vi "performanceCalc.vi"(0 "errors":dbl[](array[numeric]), 1 "init":bool, 2 "windowLength":dbl, 5 "pckTotalTrack":dbl[](array[numeric]), 7 "state":dbl[](array[numeric]), 9 "pckSuccess":dbl, 11 "pckTotal":dbl, 12 "delay":dbl) -> (4 "errorsOut":dbl[](array[numeric]), 6 "pckTotalTrackOut":dbl[](array[numeric]), 8 "prevState":dbl[](array[numeric]))   [LabVIEW 2010]
uses:
  <vilib>/imath/engines/lvmath2/RunTimeEngine/ErrorHandling/NIMS_Finalize Error.vi
  <vilib>/imath/engines/lvmath2/RunTimeEngine/VariableToken/Read/NIMS_Get Elements - RV(_) - Check.vi
  <instcachedir>/0/NIMS_Get Elements - RV(_) - Check_1F6F8656162345078B1D4DC9877DFAE9.lvgen/NIMS_Get Elements - RV(_) - Check_1F6F8656162345078B1D4DC9877DFAE9_000.vi
  <vilib>/imathl/engines/lvmath/Functions/Error Handling/Create Error.vi
  <vilib>/imath/engines/lvmath2/RunTimeEngine/NodeEndStatement/NIMS_NodeEndStatement_Output.vi
  <instcachedir>/0/NIMS_NodeEndStatement_Output_53EC0D466D134D7ABD903AC30B43404B.lvgen/NIMS_NodeEndStatement_Output_53EC0D466D134D7ABD903AC30B43404B_001.vi
  <instcachedir>/0/NIMS_NodeEndStatement_Output_53EC0D466D134D7ABD903AC30B43404B.lvgen/NIMS_NodeEndStatement_Output_53EC0D466D134D7ABD903AC30B43404B_005.vi
  <vilib>/imath/engines/lvmath2/RunTimeEngine/BuiltInFunctions/mod/NIMS_mod_no_size_check.vi
  <instcachedir>/0/NIMS_mod_no_size_check_5393E3382FD241D281EEB71DA286C65B.lvgen/NIMS_mod_no_size_check_5393E3382FD241D281EEB71DA286C65B_001.vi
  <vilib>/imath/engines/lvmath2/RunTimeEngine/ReplaceToken/NIMS_Replace - Check(_) Linear.vi
  <instcachedir>/0/NIMS_Replace - Check(_) Linear_D531E313C4004E3DB8F0EA3CE86AE758.lvgen/NIMS_Replace - Check(_) Linear_D531E313C4004E3DB8F0EA3CE86AE758_006.vi
  <vilib>/imath/engines/lvmath2/RunTimeEngine/ReplaceToken/NIMS_Replace - Size Check _(_)=S.vi
  <instcachedir>/0/NIMS_Replace - Size Check _(_)=S_6CAC13ACC74349C582FDAB09BCDAB70F.lvgen/NIMS_Replace - Size Check _(_)=S_6CAC13ACC74349C582FDAB09BCDAB70F_000.vi
  <vilib>/imath/engines/lvmath2/RunTimeEngine/ReplaceToken/NIMS_Replace - V(S)=S.vi
  <instcachedir>/0/NIMS_Replace - V(S)=S_78FDB6CCD265407D8926E4CF958018EB.lvgen/NIMS_Replace - V(S)=S_78FDB6CCD265407D8926E4CF958018EB_000.vi
  <vilib>/imath/engines/lvmath2/RunTimeEngine/VariableToken/Read/NIMS_Get Elements - RV(_) - Check(_).vi
  <instcachedir>/0/NIMS_Get Elements - RV(_) - Check(_)_260A45C9C4AF472A8F32F86A1BEF7DEE.lvgen/NIMS_Get Elements - RV(_) - Check(_)_260A45C9C4AF472A8F32F86A1BEF7DEE_000.vi
  <vilib>/imath/engines/lvmath2/RunTimeEngine/BuiltInFunctions/sum/NIMS_sum(GV).vi
  <instcachedir>/0/NIMS_sum(GV)_67F5EC36BC034E54A6BEC5B0673C00E5.lvgen/NIMS_sum(GV)_67F5EC36BC034E54A6BEC5B0673C00E5_000.vi
  <vilib>/imath/engines/lvmath2/RunTimeEngine/ReplaceToken/NIMS_Replace - Check Linear.vi
  <instcachedir>/0/NIMS_Replace - Check Linear_662D5651E4E34E0584DA82A256193A4C.lvgen/NIMS_Replace - Check Linear_662D5651E4E34E0584DA82A256193A4C_001.vi
  <vilib>/imath/engines/lvmath2/RunTimeEngine/ErrorHandling/NIMS_Create Error From Enums.vi
panel:
  out "interSampling":dbl
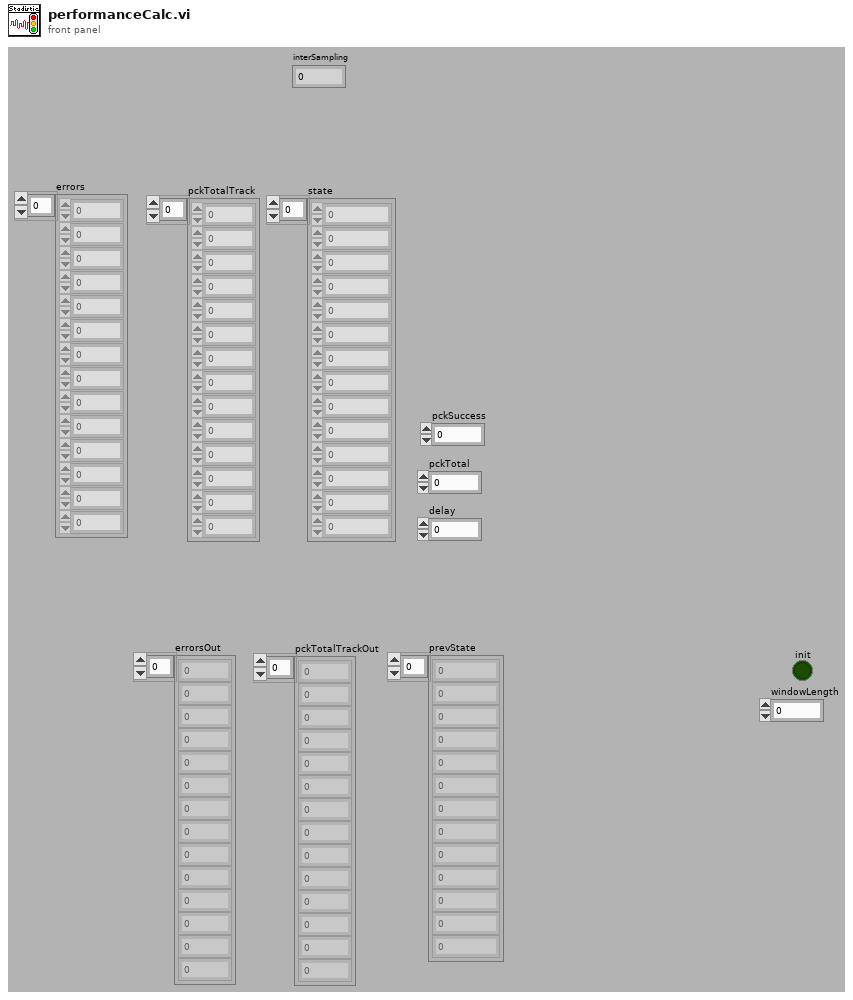
[diagram p1: front panel]
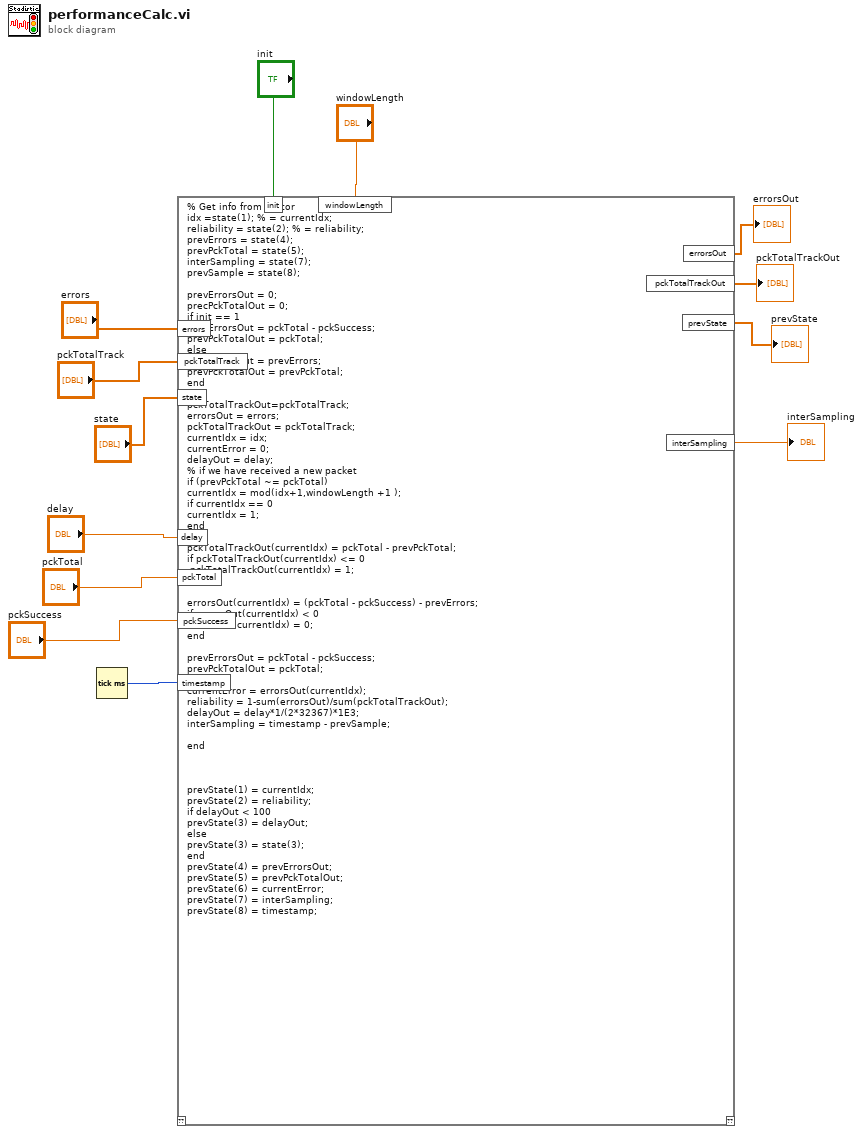
[diagram p0: block diagram]
diagram:
  n1 = Tick Count (ms)() -> (millisecond timer value=w2:u32)
  n2 = mathscript code="% Get info from vector\nidx =state(1); % = currentIdx;\nreliability = state(2); % = reliability;\nprevErrors = state(4);\nprevPckTotal = state(5);\ninterSampling = state(7);\nprevSample = state(8);\n\nprevErrorsOut = 0;\nprecPckTotalOut = 0;\nif init == 1\nprevErrorsOut = pckTotal - pckSuccess;\nprevPckTotalOut = pckTotal;\nelse\nprevErrorsOut = prevErrors;\nprevPckTotalOut = prevPckTotal;\nend\n\npckTotalTrackOut=pckTotalTrack;\nerrorsOut = errors;\npckTotalTrackOut = pckTotalTrack;\ncurrentIdx = idx;\ncurrentError = 0;\ndelayOut = delay;\n% if we have received a new packet\nif (prevPckTotal ~= pckTotal)\ncurrentIdx = mod(idx+1,windowLength +1 );\nif currentIdx == 0\ncurrentIdx = 1;\nend\n\npckTotalTrackOut(currentIdx) = pckTotal - prevPckTotal;\nif pckTotalTrackOut(currentIdx) <= 0\n pckTotalTrackOut(currentIdx) = 1;\nend\n\nerrorsOut(currentIdx) = (pckTotal - pckSuccess) - prevErrors;\nif errorsOut(currentIdx) < 0\nerrorsOut(currentIdx) = 0;\nend\n\nprevErrorsOut = pckTotal - pckSuccess;\nprevPckTotalOut = pckTotal;\n\ncurrentError = errorsOut(currentIdx);\nreliability = 1-sum(errorsOut)/sum(pckTotalTrackOut);\ndelayOut = delay*1/(2*32367)*1E3;\ninterSampling = timestamp - prevSample;\n\nend\n\n\n\nprevState(1) = currentIdx;\nprevState(2) = reliability;\nif delayOut < 100\nprevState(3) = delayOut;\nelse\nprevState(3) = state(3);\nend\nprevState(4) = prevErrorsOut;\nprevState(5) = prevPckTotalOut;\nprevState(6) = currentError;\nprevState(7) = interSampling;\nprevState(8) = timestamp;"("pckSuccess"="pckSuccess", "pckTotal"="pckTotal", "delay"="delay", "errors"="errors", "pckTotalTrack"="pckTotalTrack", "windowLength"="windowLength", "init"="init", "state"="state", "timestamp"=w2) -> ("errorsOut"=→"errorsOut":dbl[], "pckTotalTrackOut"=→"pckTotalTrackOut":dbl[], "prevState"=→"prevState":dbl[], "interSampling"=→"interSampling":dbl)  [unwired: 1 in, 1 out]
